vi "SRV_PM_Parse Packet.vi"(0 "Packet":u8[](array[numeric]) format="%.0x", 11 "error in (no error)":errorcluster, 12 "Gen Err? (T)":bool=TRUE) -> (1 "Command Type":u8[](array[numeric]) format="%.0x", 2 "Sender":u8[](array[numeric]) format="%.0x", 3 "Timestamp":u8[](array[numeric]) format="%.0x", 4 "Packet Data dup":u8[](array[numeric]) format="%.0x", 6 "Data Field Length":u16 format="%.0x", 8 "Data Field":u8[](array[numeric]) format="%.0x", 10 "Checksum":u8[](array[numeric]) format="%.0x", 13 "Packet Data sans Extra Bytes":u8[](array[numeric]) format="%.0x", 14 "Extra Bytes":u8[](array[numeric]) format="%.0x", 15 "error out":errorcluster)   [LabVIEW 2009]
panel:
  out "Data String":string
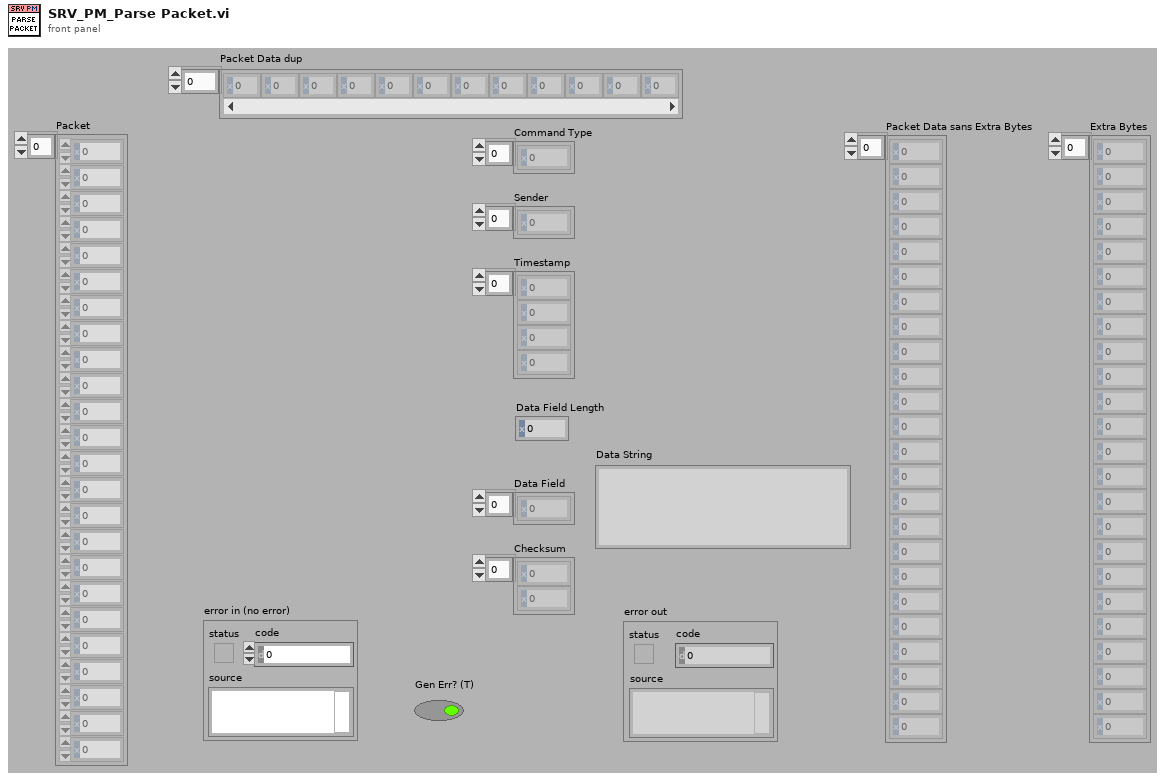
[diagram p1: front panel]
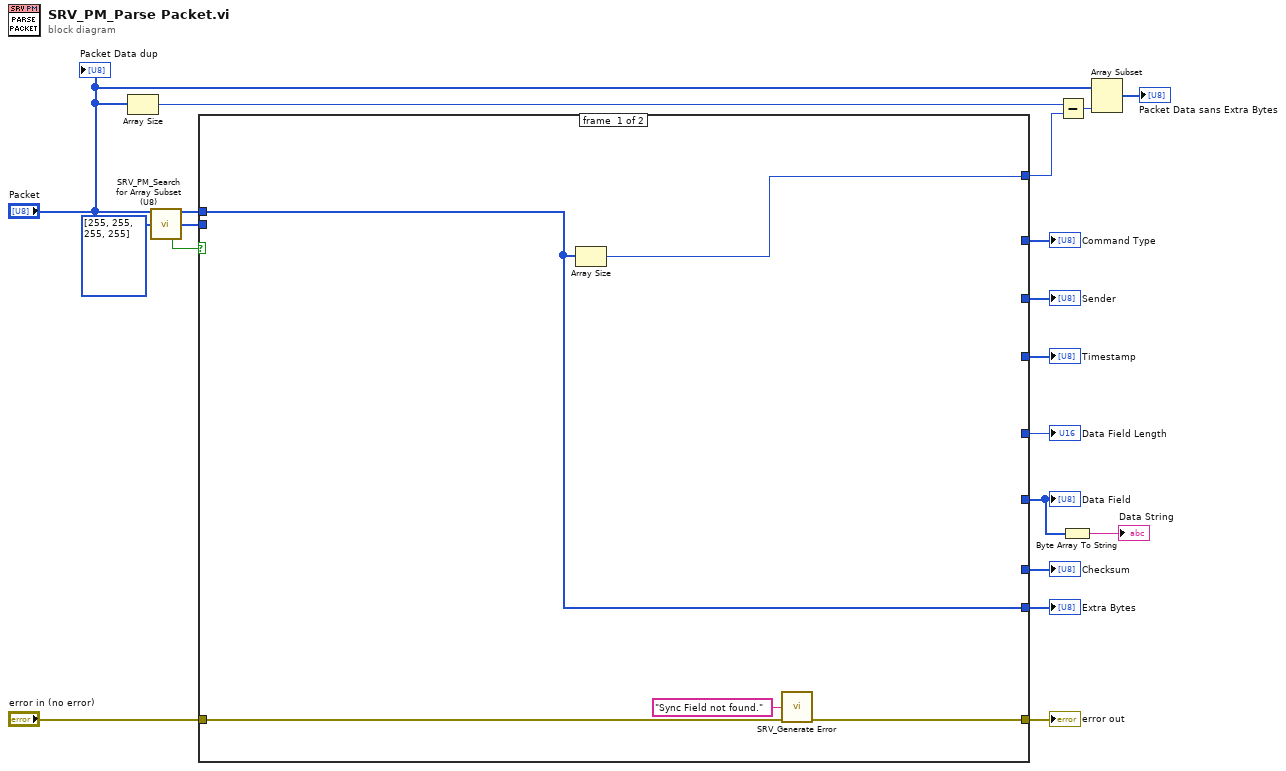
[diagram p0: block diagram]
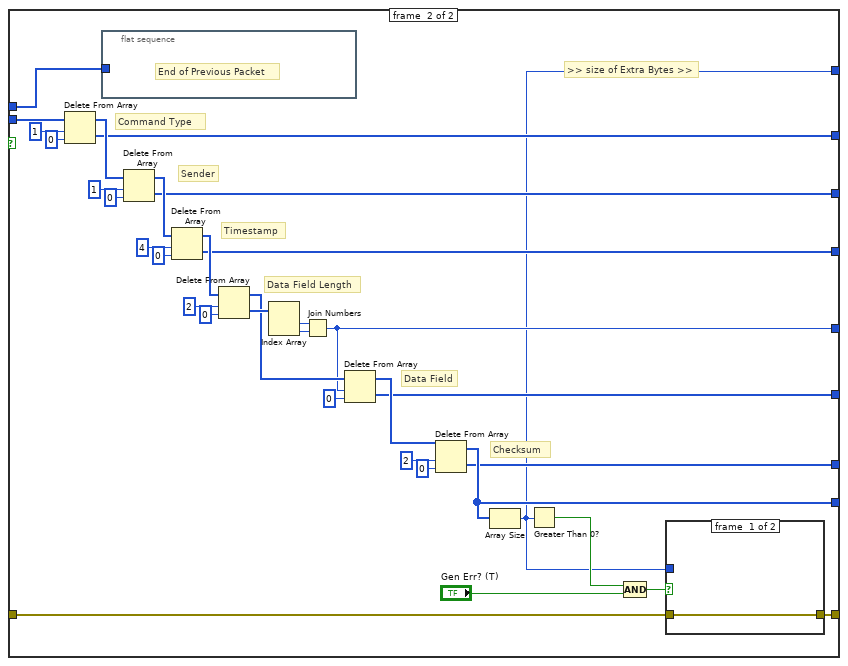
[diagram p2: hidden frame]
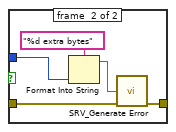
[diagram p3: hidden frame]
diagram:
  n1 = Array Size(array="Packet") -> (size(s)=w5:i32)
  n2 = call "SRV_PM_Search for Array Subset (U8).vi"("1D Array"="Packet", "Search"=u8[] [255, 255, 255, 255] ("Sync Field")) -> ("Before Match"=w17:u8[], "After Match"=w15:u8[], "Found?"=w18:bool)  [unwired: 8 in, 3 out]
  n3 = case shown="True" w18 {
    tunnel: w17 -> [w21 w58]
    tunnel: [w21 w37] -> w16
    tunnel: w15 -> [_ w57]
    tunnel: "error in (no error)" -> [w23 w36]
    tunnel: [w24 w35] -> w13
    tunnel: [_ w34] -> w12
    tunnel: [_ w33] -> w11
    tunnel: [_ w32] -> w10
    tunnel: [_ w31] -> w9
    tunnel: [_ w30] -> w7
    tunnel: [_ w29] -> w8
    tunnel: [w20 w25] -> w4
    frame #0 {
      n4 = Array Size(array=w21) -> (size(s)=w20:i32)
      n5 = call "SRV_Generate Error.vi"("Message"="Sync Field not found.", "error in (no error)"=w23) -> ("error out"=w24:errorcluster)  [unwired: 13 in]
    }
    frame #1 {
      # ">> size of Extra Bytes >>"
      # "Checksum"
      # "Data Field"
      # "Data Field Length"
      # "Timestamp"
      # "Sender"
      # "Command Type"
      n6 = Delete From Array(array=w57, length=1, index=0) -> (deleted portion=w34:u8[], array with subset deleted=w52:u8[])
      n7 = flat-sequence {
        tunnel: w58 -> [_]
        frame #0 {
          # "End of Previous Packet"
        }
      }
      n8 = Delete From Array(array=w52, length=1, index=0) -> (deleted portion=w33:u8[], array with subset deleted=w49:u8[])
      n9 = Delete From Array(array=w49, length=4, index=0) -> (deleted portion=w32:u8[], array with subset deleted=w46:u8[])
      n10 = Delete From Array(array=w46, length=2, index=0) -> (deleted portion=w45:u8[], array with subset deleted=w41:u8[])
      n11 = Index Array(array=w45) -> (element #1=w44:u8, element #2=w43:u8)  [unwired: 2 in]
      n12 = Join Numbers(hi=w44, lo=w43) -> ((hi.lo)=w31:u16)
      n13 = Delete From Array(array=w41, length=w31, index=0) -> (deleted portion=w30:u8[], array with subset deleted=w40:u8[])
      n14 = Delete From Array(array=w40, length=2, index=0) -> (deleted portion=w29:u8[], array with subset deleted=w37:u8[])
      n15 = Array Size(array=w37) -> (size(s)=w25:i32)
      n16 = Greater Than 0?(x=w25) -> (x > 0?=w28:bool)
      n17 = Compound Arithmetic op=AND(w28, "Gen Err? (T)") -> (w26:bool)
      n18 = case shown="True" w26 {
        tunnel: w36 -> [w59 w64]
        tunnel: [w59 w63] -> w35
        tunnel: w25 -> [_ w60]
        frame #0 {
        }
        frame #1 {
          n19 = Format Into String(format string="%d extra bytes", w60) -> (resulting string=w61:string)  [unwired: 2 in, 1 out]
          n20 = call "SRV_Generate Error.vi"("Message"=w61, "error in (no error)"=w64) -> ("error out"=w63:errorcluster)  [unwired: 13 in]
        }
      }
    }
  }
  "error out" <- w13
  "Extra Bytes" <- w16
  "Command Type" <- w12
  "Sender" <- w11
  "Timestamp" <- w10
  "Data Field Length" <- w9
  "Data Field" <- w7
  "Checksum" <- w8
  n21 = Subtract(x=w5, y=w4) -> (x-y=w3:i32)
  n22 = Byte Array To String(unsigned byte array=w7) -> (string=→"Data String":string)
  n23 = Array Subset(array="Packet", length=w3) -> (→"Packet Data sans Extra Bytes":u8[])  [unwired: 1 in]
  "Packet Data dup" <- "Packet"
